vi "FormingTR_DQ.vi"(2 "TranslationVector":dbl[](array[numeric]), 3 "UnitVectorAxis":dbl[](array[numeric]), 4 "Theta(D)":dbl) -> (0 "R":dbl[](array[numeric]), 1 "TR_DQ":cluster{"q":T1, "qe":T1})   [LabVIEW 2014]
doc: "用对偶四元数的TR形式实现图片的3D运动"
uses:
  <vilib>/robotics/Kinematics/Quaternion.ctl
  <vilib>/robotics/Kinematics/Multiply Quaternion by Quaternion.vi
  <vilib>/robotics/Kinematics/NI_Kinematics.lvlib
panel:
  out "v'":cluster{"q":T1, "qe":T1}
  in  "v":cluster{"q":T1, "qe":T1}={"q"=[1.0, 0.0, 0.0, 0.0], "qe"=[]}
  # "rotation followed by translation"
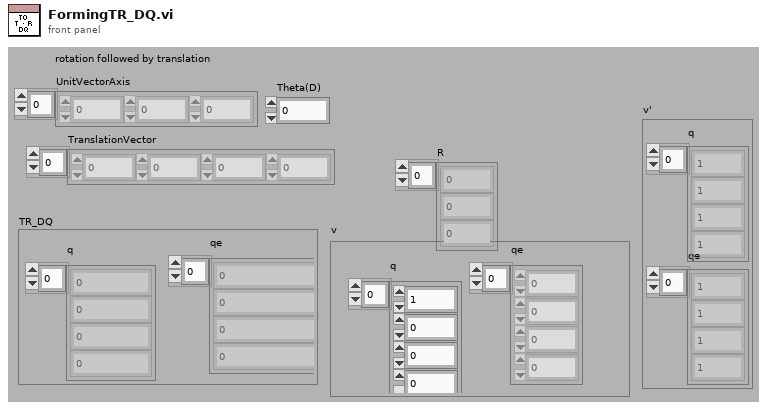
[diagram p1: front panel]
types:
  T1 = typedef "NI_Kinematics.lvlib/Quaternion.ctl" = dbl[]
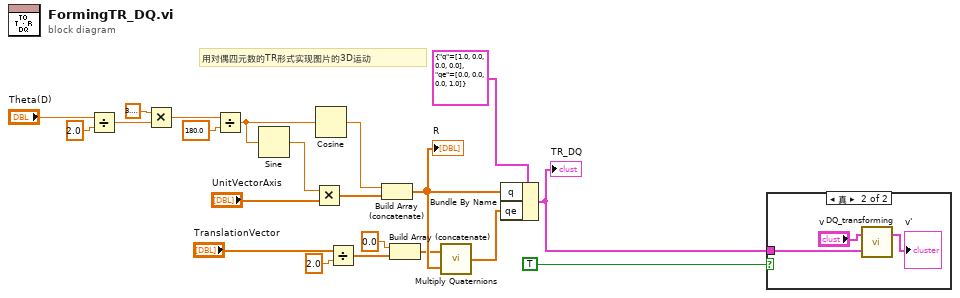
[diagram p0: block diagram]
diagram:
  # "用对偶四元数的TR形式实现图片的3D运动"
  n1 = Divide(x="Theta(D)", y=2.0) -> (x/y=w19:dbl)
  n2 = Multiply(x=3.141592653589793, y=w19) -> (x*y=w14:dbl)
  n3 = Divide(x=w14, y=180.0) -> (x/y=w13:dbl)
  n4 = Sine(x=w13) -> (sin(x)=w11:dbl)
  n5 = Multiply(x=w11, y="UnitVectorAxis") -> (x*y=w17:dbl[])
  n6 = Cosine(x=w13) -> (cos(x)=w16:dbl)
  n7 = Divide(x="TranslationVector", y=2.0) -> (x/y=w8:dbl[])
  n8 = Build Array (concatenate) ("创建数组")(w16, w17) -> (w3:dbl[])
  "R" <- w3
  n9 = Build Array (concatenate)(0.0 ("Numeric"), w8) -> (w2:dbl[])
  n10 = call-poly <vilib>:"Multiply Quaternions.vi"("y"=w3, "quaternion"=w2) -> ("product"=w7:T1)
  n11 = Bundle By Name(cluster=cluster{"q":T1, "qe":T1} {"q"=[1.0, 0.0, 0.0, 0.0], "qe"=[0.0, 0.0, 0.0, 1.0]} ("Vector"), "q"=w3, "qe"=w7) -> (w1:cluster{"q":T1, "qe":T1})
  "TR_DQ" <- w1
  n12 = case shown="真" TRUE {
    tunnel: w1 -> [_ w24]
    frame False {
    }
    frame True {
      n13 = call "DQ_transforming.vi"("DQ"=w24, "Vector"="v") -> ("transformedVector"=→"v'":cluster{"q":T1, "qe":T1})  [unwired: 1 out]
    }
  }
